vi "AD420_SPI_Digital_output.vi"() -> ()   [LabVIEW 2015]
uses:
  <vilib>/myRIO/Instrument Drivers/Onboard IO/DIO/typedefs/DIO Reference.ctl
  <vilib>/myRIO/Common/Instrument Driver Framework/Utilities/typedefs/myRIO Generic Hardware Reference.ctl
  <vilib>/myRIO/Common/Instrument Driver Framework/Utilities/typedefs/Hardware Version Enum.ctl
  <vilib>/myRIO/Common/Instrument Driver Framework/Utilities/typedefs/myRIO v1.0 Reference.ctl
  <vilib>/myRIO/Common/Instrument Driver Framework/Utilities/typedefs/Generic FPGA Reference.ctl
  <vilib>/myRIO/Common/Instrument Driver Framework/myRIO v1.0/DIO/typedefs/DIO Channels List.ctl
  <vilib>/myRIO/Common/Instrument Driver Framework/myRIO v1.0/DIO/typedefs/DIO Channels Enum.ctl
  <vilib>/userdefined/High Color/nirio_resource_hc.ctl
  <vilib>/myRIO/Common/Instrument Driver Framework/Utilities/vis/Is FPGA Ref Available.vi
  <vilib>/myRIO/Common/Instrument Driver Framework/myRIO v1.0/DIO/vis/myRIO v1.1 Open DIO.vi
  <vilib>/myRIO/Instrument Drivers/Onboard IO/DIO/vis/Write.vi
  <vilib>/myRIO/Common/Instrument Driver Framework/Utilities/vis/Validate Channels.vi
  <vilib>/myRIO/Common/Instrument Driver Framework/myRIO v1.0/DIO/vis/myRIO v1.0 Reserve DIO.vi
  <vilib>/myRIO/Common/Instrument Driver Framework/myRIO v1.0/Resource Manager/vis/myRIO v1.0 Reserve Channel List.vi
  <vilib>/myRIO/Common/Instrument Driver Framework/myRIO v1.0/DIO/vis/myRIO v1.0 Build MUX Configuration DIO.vi
  <vilib>/myRIO/Common/Instrument Driver Framework/myRIO v1.0/Resource Manager/vis/myRIO v1.0 Reserve Channel.vi
  <vilib>/myRIO/Common/Instrument Driver Framework/myRIO v1.0/Resource Manager/vis/myRIO v1.0 Unreserve Channel.vi
  <vilib>/myRIO/Common/Instrument Driver Framework/myRIO v1.0/Resource Manager/vis/myRIO v1.0 Create Configuration List.vi
  <vilib>/myRIO/Common/Instrument Driver Framework/myRIO v1.0/Resource Manager/vis/myRIO v1.0 Build Mutex Name.vi
  <vilib>/Utility/VariantDataType/GetNumericInfo.vi
  <vilib>/Utility/error.llb/Error Cluster From Error Code.vi
  <vilib>/myRIO/Common/Instrument Driver Framework/myRIO v1.0/myRIO v1.1 Open.vi
  <vilib>/myRIO/Common/Instrument Driver Framework/Utilities/vis/IO Manager.vi
  <vilib>/myRIO/Common/Instrument Driver Framework/Utilities/vis/Configuration Manager.vi
  <vilib>/myRIO/Common/Instrument Driver Framework/myRIO v1.0/Resource Manager/vis/myRIO v1.0 Configure IO.vi
  <vilib>/myRIO/Common/Instrument Driver Framework/myRIO v1.0/myRIO v1.0 Close.vi
  <vilib>/myRIO/Common/Instrument Driver Framework/myRIO v1.0/DIO/vis/myRIO v1.0 Write DIO.vi
  <vilib>/myRIO/Express VI/Onboard IO/DO/DO Express VI.xnode
  <vilib>/myRIO/Instrument Drivers/Onboard IO/DIO/vis/myRIO DIO Open.xnode
  <vilib>/myRIO/Instrument Drivers/Onboard IO/DIO/DIO.lvlib
panel:
  out "Decimal equivalent":dbl
  out "Binary equivalent":i16[](array[numeric])
  in  "Voltage":dbl min=-10.0 max=10.0
  # "Request your voltage here"
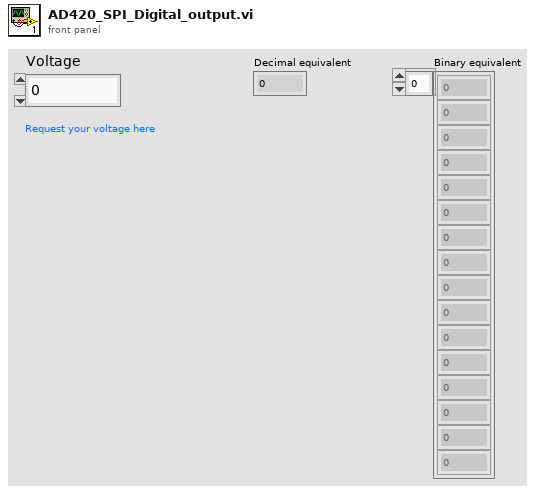
[diagram p1: front panel]
types:
  T1 = typedef "DIO.lvlib/DIO Reference.ctl" = cluster{"myRIO Reference":T2, "DIO Channels List":T6}
  T2 = typedef "myRIO Generic Hardware Reference.ctl" = cluster{"myRIO Model":T3, "myRIO Hardware Reference":T4}
  T3 = typedef "Hardware Version Enum.ctl" = enum16{"Unknown", "myRIO-1900", "myRIO-1950", "roboRIO"}
  T4 = typedef "myRIO v1.0 Reference.ctl" = cluster{"Generic FPGA Reference":T5, "Allow multiple opens":bool}
  T5 = typedef "Generic FPGA Reference.ctl" = refnum<k20>
  T6 = typedef "DIO Channels List.ctl" = T7[]
  T7 = typedef "DIO Channels Enum.ctl" = enum16{"Not Connected", "C/DIO0", "C/DIO1", "C/DIO2", "C/DIO3", "C/DIO4", "C/DIO5", "C/DIO6", "C/DIO7", "A/DIO0", "A/DIO1", "A/DIO2", "A/DIO3", "A/DIO4", "A/DIO5", "A/DIO6", "A/DIO7", "A/DIO8", "A/DIO9", "A/DIO10", "A/DIO11", "A/DIO12", "A/DIO13", "A/DIO14", "A/DIO15", "B/DIO0", "B/DIO1", "B/DIO2", "B/DIO3", "B/DIO4", "B/DIO5", "B/DIO6", "B/DIO7", "B/DIO8", "B/DIO9", "B/DIO10", "B/DIO11", "B/DIO12", "B/DIO13", "B/DIO14", "B/DIO15", "LED0", "LED1", "LED2", "LED3", "Button0", "DIO/DIO0", "DIO/DIO1", "DIO/DIO2", "DIO/DIO3", "DIO/DIO4", "DIO/DIO5", "DIO/DIO6", "DIO/DIO7", "DIO/DIO8", "DIO/DIO9", "SPI/CS0", "SPI/CS1", "SPI/CS2", "SPI/CS3", "LED RADIO (Green)", "LED RADIO (Red)", "LED COMM (Green)", "LED COMM (Red)", "LED MODE (Green)", "LED MODE (Red)"}
  T8 = typedef "nirio_resource_hc.ctl" = tag
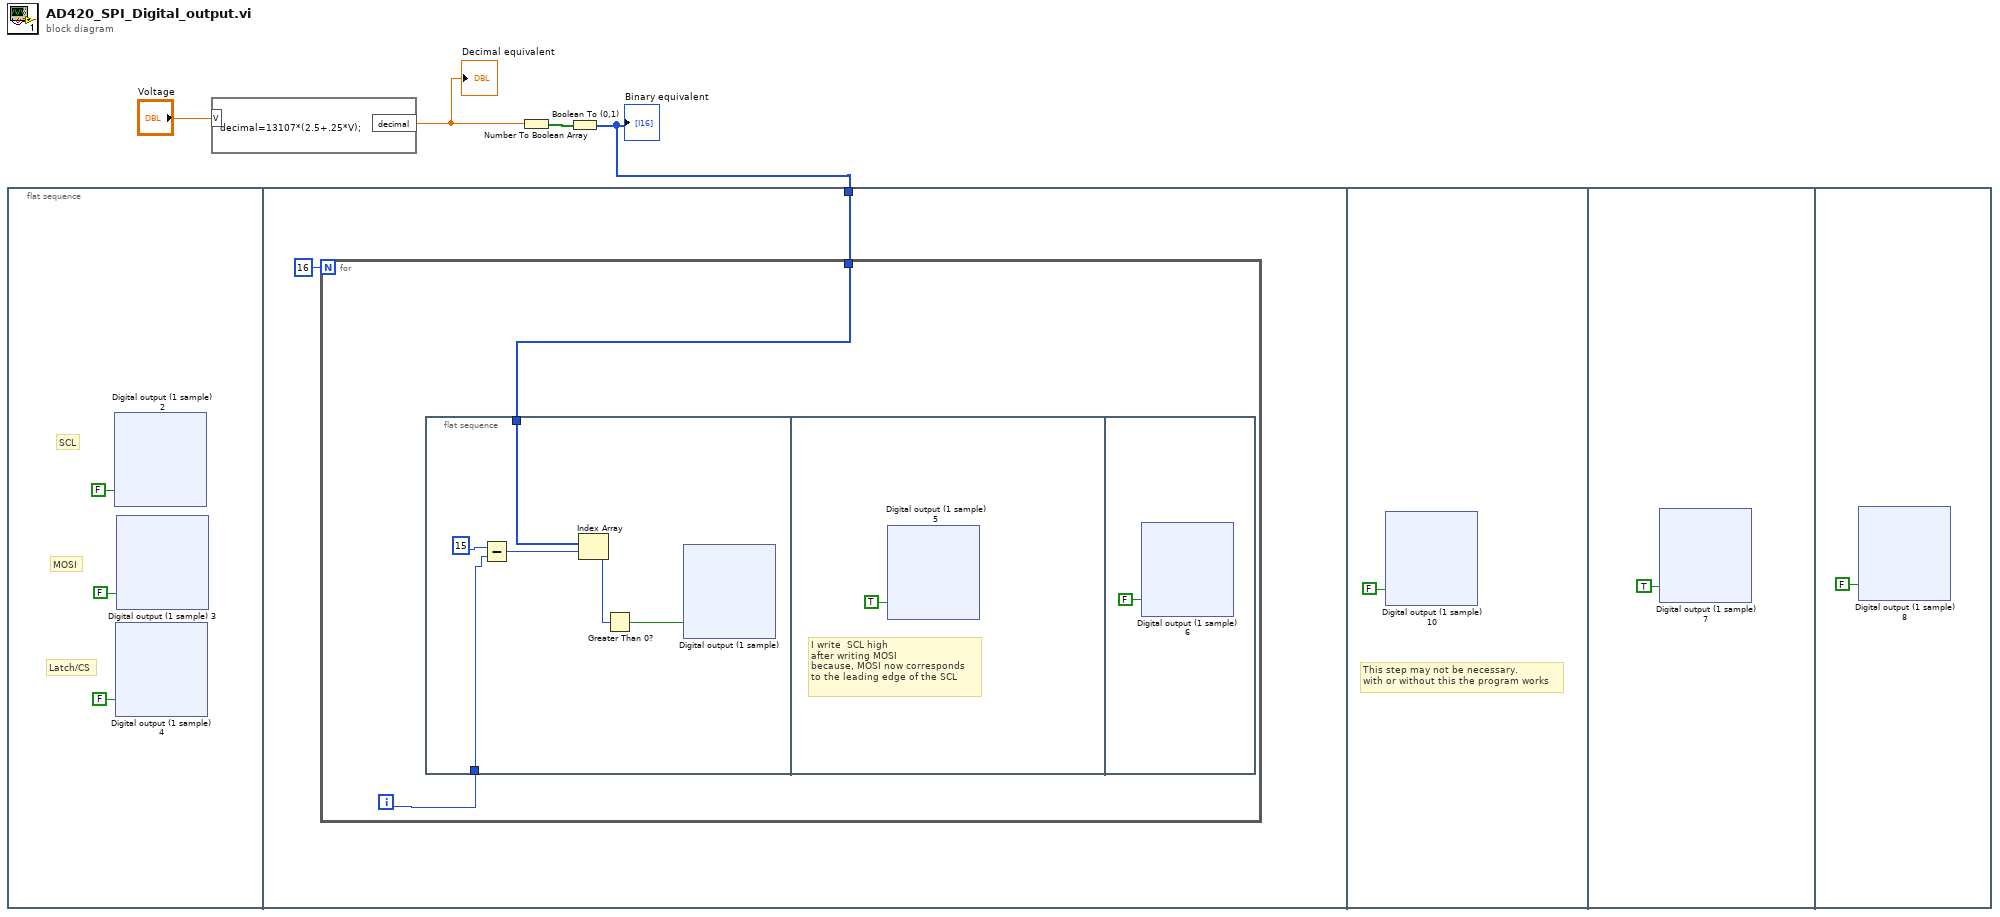
[diagram p0: block diagram]
diagram:
  n1 = flat-sequence {
    tunnel: w1 -> [w114]
    frame #0 {
      # "Latch/CS"
      # "MOSI"
      # "SCL"
      n2 = xnode "Digital output (1 sample) 2"("A/DIO0 (Pin 11)"=FALSE ("A/DIO1 (Pin 13)")) -> ()  [unwired: 1 in, 1 out]
      n3 = xnode "Digital output (1 sample) 4"("A/DIO2 (Pin 15)"=FALSE ("A/DIO1 (Pin 13)")) -> ()  [unwired: 1 in, 1 out]
      n4 = xnode "Digital output (1 sample) 3"("A/DIO1 (Pin 13)"=FALSE) -> ()  [unwired: 1 in, 1 out]
    }
    frame #1 {
      n5 = for {
        N: 16 -> [_]
        tunnel: w114 -> [w115]
        i -> [w116]
        n6 = flat-sequence {
          tunnel: w116 -> [w119]
          tunnel: w115 -> [w118]
          frame #0 {
            n7 = Subtract(x=15, y=w119) -> (x-y=w121:i32)
            n8 = Index Array(array=w118, index=w121) -> (element=w117:i16)
            n9 = Greater Than 0?(x=w117) -> (x > 0?=w122:bool)
            n10 = xnode "Digital output (1 sample)"("A/DIO1 (Pin 13)"=w122) -> ()  [unwired: 1 in, 1 out]
          }
          frame #1 {
            # "I write  SCL high\nafter writing MOSI \nbecause, MOSI now corresponds \nto the leading edge of the SCL"
            n11 = xnode "Digital output (1 sample) 5"("A/DIO0 (Pin 11)"=TRUE) -> ()  [unwired: 1 in, 1 out]
          }
          frame #2 {
            n12 = xnode "Digital output (1 sample) 6"("A/DIO0 (Pin 11)"=FALSE) -> ()  [unwired: 1 in, 1 out]
          }
        }
      }
    }
    frame #2 {
      # "This step may not be necessary.\nwith or without this the program works"
      n13 = xnode "Digital output (1 sample) 10"("A/DIO1 (Pin 13)"=FALSE) -> ()  [unwired: 1 in, 1 out]
    }
    frame #3 {
      n14 = xnode "Digital output (1 sample) 7"("A/DIO2 (Pin 15)"=TRUE ("A/DIO1 (Pin 13)")) -> ()  [unwired: 1 in, 1 out]
    }
    frame #4 {
      n15 = xnode "Digital output (1 sample) 8"("A/DIO2 (Pin 15)"=FALSE ("A/DIO1 (Pin 13)")) -> ()  [unwired: 1 in, 1 out]
    }
  }
  n16 = formula code="decimal=13107*(2.5+.25*V);"("V"="Voltage") -> ("decimal"=w2:dbl)
  "Decimal equivalent" <- w2
  n17 = Number To Boolean Array(number=w2) -> (Boolean array=w3:bool[])
  n18 = Boolean To (0,1)(Boolean=w3) -> (0, 1=w1:i16[])
  "Binary equivalent" <- w1
